vi "Autonomous Independent.vi"() -> ()   [LabVIEW 2017]
doc: "This VI is called when autonomous begins, and will automatically be terminated when autonomous ends. You can carry out timed or sensor driven robot movement independently without needing to return to the caller."
uses:
  <vilib>/Rock Robotics/WPI/RobotDrive/WPI_RobotDriveMecanumDrive_Cartesian.vi
  Robot Global Data.vi
  <vilib>/Rock Robotics/WPI/ThirdParty/Sensors/ADIS16448 IMU/ADIS16448_IMU.lvlib
  <vilib>/Rock Robotics/Network Tables/NT Read String.vi
panel:
  in  "secondTurnAngle":dbl
  in  "distPinceHigh":dbl
  in  "pinceRaiseSpeed":dbl
  in  "pinceLowerSpeed":dbl
  in  "distPinceLow 1":dbl
  in  "angleWall":dbl=-48.0
  in  "angleFloor":dbl=-2.0
  in  "angleRamp":dbl=-7.0
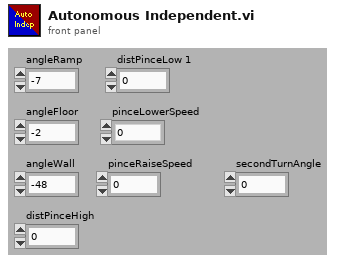
[diagram p1: front panel]
types:
  T1 = typedef "WPI_RobotDriveDevRef.ctl" = cluster{"DevStatus":errorcluster, "Motors[]":T2[], "Square Inputs":bool, "Max Output":dbl}
  T2 = typedef "WPI_MotorControlDeviceRef.ctl" = cluster{"DeviceStatus":errorcluster, "Type":T3, "PWM":cluster{"PWM Channel":T4, "DeadBand":T5}, "CAN":cluster{"Device Number":u8, "SetOutput VI Ref":variant, "GetOutput VI Ref":variant, "Enable VI Ref":variant, "Disable VI Ref":variant, "Data":variant}, "Invert":bool, "DIO PWM":cluster{"PWM \"Enable\" Channel":T4, "DIOChannel":T6, "PWM Rate":dbl}}
  T3 = typedef "WPI_MotorControlType.ctl" = enum16{"PWM", "CAN", "DIO PWM"}
  T4 = typedef "FPGA_DIOPWMChannel.ctl" = enum8{"PWM 0", "PWM 1", "PWM 2", "PWM 3", "PWM 4", "PWM 5", "PWM 6", "PWM 7", "PWM 8", "PWM 9", "PWM MXP 0", "PWM MXP 1", "PWM MXP 2", "PWM MXP 3", "PWM MXP 4", "PWM MXP 5", "PWM MXP 6", "PWM MXP 7", "PWM MXP 8", "PWM MXP 9", "Invalid"}
  T5 = typedef "WPI_PWMDeadband.ctl" = cluster{"Name":string, "maxPositivePwm":i32, "minPositivePwm":i32, "centerPwm":i32, "maxNegativePwm":i32, "minNegativePwm":i32, "angularRange":u16}
  T6 = typedef "FPGA_DIOChannel.ctl" = enum8{"DIO 0", "DIO 1", "DIO 2", "DIO 3", "DIO 4", "DIO 5", "DIO 6", "DIO 7", "DIO 8", "DIO 9", "DIO MXP 0", "DIO MXP 1", "DIO MXP 2", "DIO MXP 3", "DIO MXP 4", "DIO MXP 5", "DIO MXP 6", "DIO MXP 7", "DIO MXP 8", "DIO MXP 9", "DIO MXP 10", "DIO MXP 11", "DIO MXP 12", "DIO MXP 13", "DIO MXP 14", "DIO MXP 15", "SPI Port CS1", "SPI Port CS2", "SPI Port CS3", "SPI Port MISO", "SPI Port MOSI", "Invalid"}
  T7 = typedef "ADIS16448_IMU.lvlib/ADI_IMU_ADIS16448_IMUDevRef.ctl" = cluster{"DevStatus":errorcluster, "Handle":i32, "SPI Bus":T8, "Device Found":bool, "Device Ready":bool, "Yaw Axis":enum16{"X", "Y", "Z"}, "AHRS Algorithm":enum16{"Complementary", "Madgwick"}, "Serial":u16, "Lot ID 2":u16, "Lot ID 1":u16, "Bytes Per Sample":u16, "Calibrate On Open?":bool}
  T8 = typedef "spi_bus.ctl" = enum16{"SPI On-Board, CS0", "SPI On-Board, CS1", "SPI On-Board, CS2", "SPI On-Board, CS3", "SPI MXP", "Invalid"}
  T9 = typedef "WPI_EncoderDevRef.ctl" = cluster{"DevStatus":errorcluster, "EncoderIndex":T10, "CounterIndex":T11, "DistancePerCount":dbl, "Decoding Type":T12}
  T10 = typedef "FPGA_EncoderIdx.ctl" = enum8{"Enc 0", "Enc 1", "Enc 2", "Enc 3", "Enc 4", "Enc 5", "Enc 6", "Enc 7", "Invalid"}
  T11 = typedef "FPGA_CounterCtrSystemIndex.ctl" = enum8{"Ctr 0", "Ctr 1", "Ctr 2", "Ctr 3", "Ctr 4", "Ctr 5", "Ctr 6", "Ctr 7", "Invalid"}
  T12 = typedef "WPI_EncoderType.ctl" = enum16{"1x", "2x", "4x"}
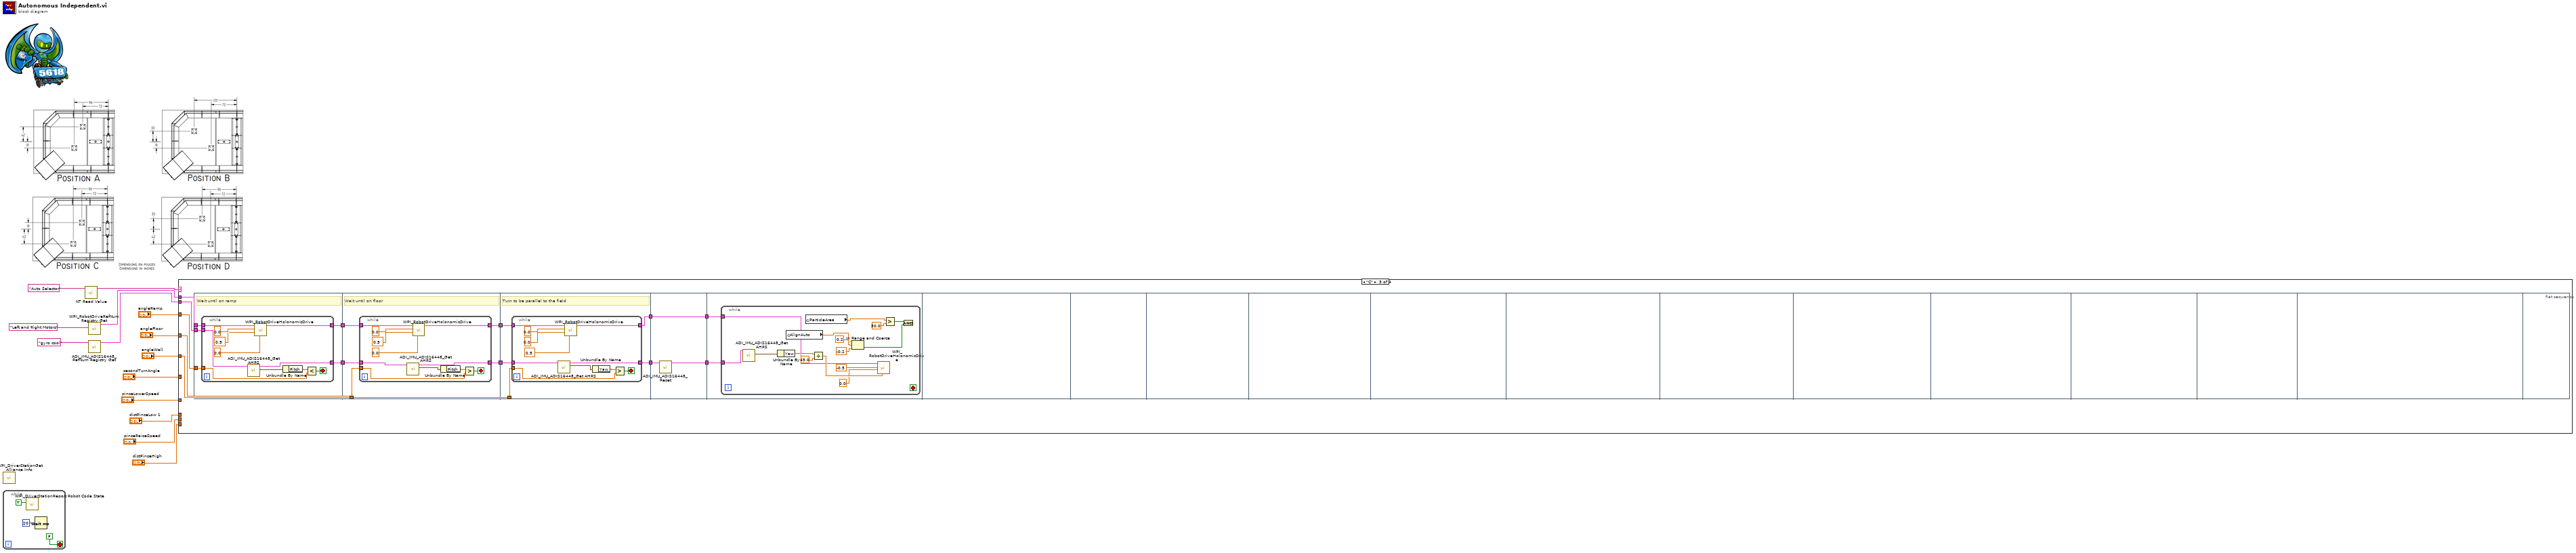
[diagram p0: block diagram]
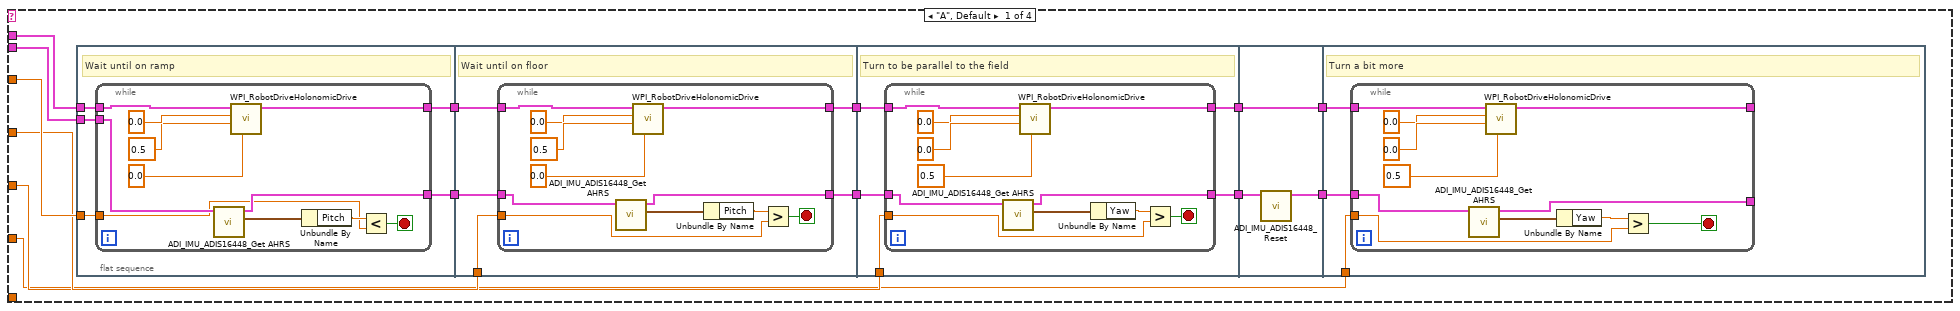
[diagram p2: hidden frame]
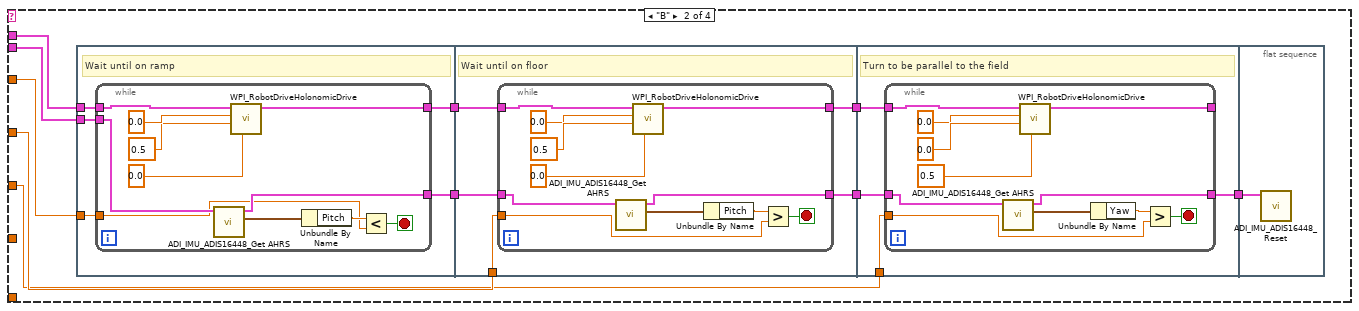
[diagram p3: hidden frame]
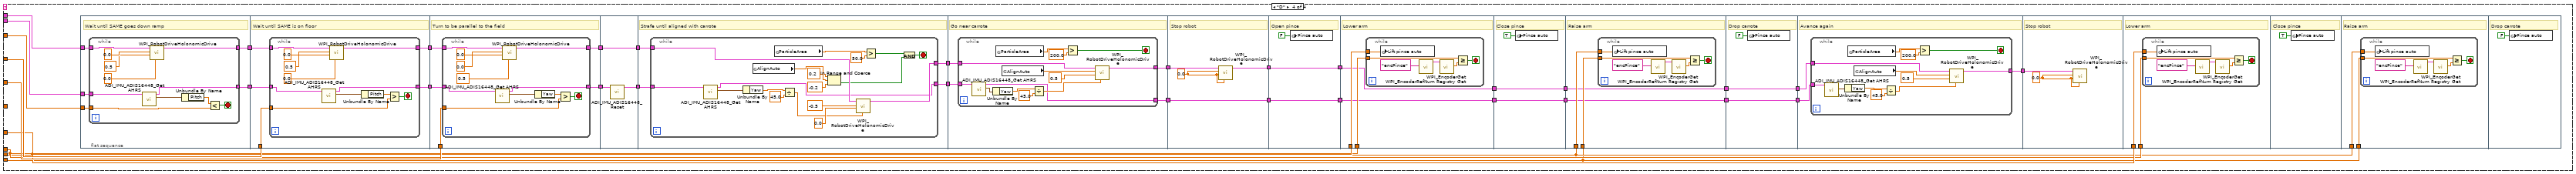
[diagram p4: hidden frame]
diagram:
  n1 = call <vilib>:"WPI_DriverStationGet Alliance Info.vi"() -> ()  [unwired: 12 out]
  n2 = while {
    stop <- FALSE stop-if-true
    n3 = call <vilib>:"WPI_DriverStationReport Robot Code State.vi"("Autonomous"=TRUE) -> ()  [unwired: 10 in, 1 out]
    n4 = Wait (ms)(milliseconds to wait=u32 20) -> ()  [unwired: 1 out]
  }
  n5 = call-poly <vilib>:"NT Read Value.vi"("Name"="Auto Selector") -> ("String"=w13:string)  [unwired: 9 in, 1 out]
  n6 = call <vilib>:"WPI_RobotDriveRefNum Registry Get.vi"("refnum name"="Left and Right Motors") -> ("RobotDriveDevRef"=w11:T1)  [unwired: 9 in, 1 out]
  n7 = call <vilib>:"ADI_IMU_ADIS16448_RefNum Registry Get.vi"("refnum name"="gyro cool") -> ("ADI IMU DevRef"=w9:T7)  [unwired: 9 in, 1 out]
  n8 = case shown="\"C\"" w13 {
    tunnel: w11 -> [w29 w102 w163 w269]
    tunnel: w9 -> [w30 w101 w162 w266]
    tunnel: "angleRamp" -> [w31 w100 w161 w261]
    tunnel: "angleFloor" -> [w28 w99 w160 w260]
    tunnel: "angleWall" -> [w25 w98 w159 w259]
    tunnel: "distPinceLow 1" -> [_ _ _ w243]
    tunnel: "pinceLowerSpeed" -> [_ _ _ w244]
    tunnel: "pinceRaiseSpeed" -> [_ _ _ w242]
    tunnel: "distPinceHigh" -> [_ _ _ w241]
    tunnel: "secondTurnAngle" -> [w18 _ _ _]
    frame "A", Default {
      n9 = flat-sequence {
        tunnel: w31 -> [w36]
        tunnel: w30 -> [w35]
        tunnel: w29 -> [w34]
        tunnel: [w33] -> w27
        tunnel: [w32] -> w26
        tunnel: w28 -> [w52]
        tunnel: w27 -> [w51]
        tunnel: w26 -> [w50]
        tunnel: [w49] -> w24
        tunnel: [w48] -> w23
        tunnel: w25 -> [w68]
        tunnel: w24 -> [w67]
        tunnel: w23 -> [w66]
        tunnel: [w65] -> w22
        tunnel: [w64] -> w19
        tunnel: w22 -> [w82]
        tunnel: [w81] -> w21
        tunnel: [w80] -> w20
        tunnel: w19 -> [w80]
        tunnel: w21 -> [w85]
        tunnel: w20 -> [w84]
        tunnel: w18 -> [w83]
        frame #0 {
          # "Wait until on ramp"
          n10 = while {
            tunnel: w34 -> [w47]
            tunnel: [w43] -> w33
            tunnel: w35 -> [w41]
            tunnel: [w38] -> w32
            tunnel: w36 -> [w37]
            stop <- w39 stop-if-true
            n11 = call <vilib>:"ADI_IMU_ADIS16448_Get AHRS.vi"("ADI IMU DevRef"=w41) -> ("IMU AHRS Out"=w42:cluster{"Pitch":dbl, "Roll":dbl, "Yaw":dbl}, "ADI IMU DevRef Out"=w38:T7)  [unwired: 7 in, 2 out]
            n12 = call-poly <vilib>:"WPI_RobotDriveHolonomicDrive.vi"("Rotation"=0.0, "Y"=0.5, "X"=0.0, "RobotDriveDevRef"=w47) -> ("RobotDriveDevRef"=w43:T1)  [unwired: 5 in, 2 out]
            n13 = Unbundle By Name(w42) -> ("Pitch"=w40:dbl)
            n14 = Less?(x=w40, y=w37) -> (x < y?=w39:bool)
          }
        }
        frame #1 {
          # "Wait until on floor"
          n15 = while {
            tunnel: w51 -> [w60]
            tunnel: [w59] -> w48
            tunnel: w50 -> [w56]
            tunnel: [w54] -> w49
            tunnel: w52 -> [w53]
            stop <- w55 stop-if-true
            n16 = call <vilib>:"ADI_IMU_ADIS16448_Get AHRS.vi"("ADI IMU DevRef"=w56) -> ("IMU AHRS Out"=w58:cluster{"Pitch":dbl, "Roll":dbl, "Yaw":dbl}, "ADI IMU DevRef Out"=w54:T7)  [unwired: 7 in, 2 out]
            n17 = call-poly <vilib>:"WPI_RobotDriveHolonomicDrive.vi"("Rotation"=0.0, "Y"=0.5, "X"=0.0, "RobotDriveDevRef"=w60) -> ("RobotDriveDevRef"=w59:T1)  [unwired: 5 in, 2 out]
            n18 = Unbundle By Name(w58) -> ("Pitch"=w57:dbl)
            n19 = Greater?(x=w57, y=w53) -> (0:w55:bool)
          }
        }
        frame #2 {
          # "Turn to be parallel to the field"
          n20 = while {
            tunnel: w66 -> [w78]
            tunnel: [w77] -> w64
            tunnel: w67 -> [w74]
            tunnel: [w70] -> w65
            tunnel: w68 -> [w69]
            stop <- w73 stop-if-true
            n21 = call <vilib>:"ADI_IMU_ADIS16448_Get AHRS.vi"("ADI IMU DevRef"=w74) -> ("IMU AHRS Out"=w76:cluster{"Pitch":dbl, "Roll":dbl, "Yaw":dbl}, "ADI IMU DevRef Out"=w70:T7)  [unwired: 7 in, 2 out]
            n22 = call-poly <vilib>:"WPI_RobotDriveHolonomicDrive.vi"("Rotation"=0.5, "Y"=0.0, "X"=0.0, "RobotDriveDevRef"=w78) -> ("RobotDriveDevRef"=w77:T1)  [unwired: 5 in, 2 out]
            n23 = Unbundle By Name(w76) -> ("Yaw"=w75:dbl)
            n24 = Greater?(x=w75, y=w69) -> (0:w73:bool)
          }
        }
        frame #3 {
          n25 = call <vilib>:"ADI_IMU_ADIS16448_Reset.vi"("ADI IMU DevRef"=w82) -> ("ADI IMU DevRef Out"=w81:T7)  [unwired: 9 in, 1 out]
        }
        frame #4 {
          # "Turn a bit more"
          n26 = while {
            tunnel: w84 -> [w95]
            tunnel: [w94] -> _
            tunnel: w85 -> [w91]
            tunnel: [w87] -> _
            tunnel: w83 -> [w86]
            stop <- w90 stop-if-true
            n27 = call <vilib>:"ADI_IMU_ADIS16448_Get AHRS.vi"("ADI IMU DevRef"=w91) -> ("IMU AHRS Out"=w93:cluster{"Pitch":dbl, "Roll":dbl, "Yaw":dbl}, "ADI IMU DevRef Out"=w87:T7)  [unwired: 7 in, 2 out]
            n28 = call-poly <vilib>:"WPI_RobotDriveHolonomicDrive.vi"("Rotation"=0.5, "Y"=0.0, "X"=0.0, "RobotDriveDevRef"=w95) -> ("RobotDriveDevRef"=w94:T1)  [unwired: 5 in, 2 out]
            n29 = Unbundle By Name(w93) -> ("Yaw"=w92:dbl)
            n30 = Greater?(x=w92, y=w86) -> (0:w90:bool)
          }
        }
      }
    }
    frame "B" {
      n31 = flat-sequence {
        tunnel: w100 -> [w111]
        tunnel: w101 -> [w110]
        tunnel: w102 -> [w109]
        tunnel: [w108] -> w106
        tunnel: [w107] -> w105
        tunnel: w99 -> [w127]
        tunnel: w106 -> [w126]
        tunnel: w105 -> [w125]
        tunnel: [w124] -> w104
        tunnel: [w123] -> w103
        tunnel: w98 -> [w142]
        tunnel: w104 -> [w141]
        tunnel: w103 -> [w140]
        tunnel: [w139] -> w97
        tunnel: w97 -> [w154]
        frame #0 {
          # "Wait until on ramp"
          n32 = while {
            tunnel: w109 -> [w122]
            tunnel: [w118] -> w108
            tunnel: w110 -> [w116]
            tunnel: [w113] -> w107
            tunnel: w111 -> [w112]
            stop <- w114 stop-if-true
            n33 = call <vilib>:"ADI_IMU_ADIS16448_Get AHRS.vi"("ADI IMU DevRef"=w116) -> ("IMU AHRS Out"=w117:cluster{"Pitch":dbl, "Roll":dbl, "Yaw":dbl}, "ADI IMU DevRef Out"=w113:T7)  [unwired: 7 in, 2 out]
            n34 = call-poly <vilib>:"WPI_RobotDriveHolonomicDrive.vi"("Rotation"=0.0, "Y"=0.5, "X"=0.0, "RobotDriveDevRef"=w122) -> ("RobotDriveDevRef"=w118:T1)  [unwired: 5 in, 2 out]
            n35 = Unbundle By Name(w117) -> ("Pitch"=w115:dbl)
            n36 = Less?(x=w115, y=w112) -> (x < y?=w114:bool)
          }
        }
        frame #1 {
          # "Wait until on floor"
          n37 = while {
            tunnel: w126 -> [w135]
            tunnel: [w134] -> w123
            tunnel: w125 -> [w131]
            tunnel: [w129] -> w124
            tunnel: w127 -> [w128]
            stop <- w130 stop-if-true
            n38 = call <vilib>:"ADI_IMU_ADIS16448_Get AHRS.vi"("ADI IMU DevRef"=w131) -> ("IMU AHRS Out"=w133:cluster{"Pitch":dbl, "Roll":dbl, "Yaw":dbl}, "ADI IMU DevRef Out"=w129:T7)  [unwired: 7 in, 2 out]
            n39 = call-poly <vilib>:"WPI_RobotDriveHolonomicDrive.vi"("Rotation"=0.0, "Y"=0.5, "X"=0.0, "RobotDriveDevRef"=w135) -> ("RobotDriveDevRef"=w134:T1)  [unwired: 5 in, 2 out]
            n40 = Unbundle By Name(w133) -> ("Pitch"=w132:dbl)
            n41 = Greater?(x=w132, y=w128) -> (0:w130:bool)
          }
        }
        frame #2 {
          # "Turn to be parallel to the field"
          n42 = while {
            tunnel: w140 -> [w152]
            tunnel: [w151] -> _
            tunnel: w141 -> [w148]
            tunnel: [w144] -> w139
            tunnel: w142 -> [w143]
            stop <- w147 stop-if-true
            n43 = call <vilib>:"ADI_IMU_ADIS16448_Get AHRS.vi"("ADI IMU DevRef"=w148) -> ("IMU AHRS Out"=w150:cluster{"Pitch":dbl, "Roll":dbl, "Yaw":dbl}, "ADI IMU DevRef Out"=w144:T7)  [unwired: 7 in, 2 out]
            n44 = call-poly <vilib>:"WPI_RobotDriveHolonomicDrive.vi"("Rotation"=0.5, "Y"=0.0, "X"=0.0, "RobotDriveDevRef"=w152) -> ("RobotDriveDevRef"=w151:T1)  [unwired: 5 in, 2 out]
            n45 = Unbundle By Name(w150) -> ("Yaw"=w149:dbl)
            n46 = Greater?(x=w149, y=w143) -> (0:w147:bool)
          }
        }
        frame #3 {
          n47 = call <vilib>:"ADI_IMU_ADIS16448_Reset.vi"("ADI IMU DevRef"=w154) -> ()  [unwired: 9 in, 2 out]
        }
      }
    }
    frame "C" {
      n48 = flat-sequence {
        tunnel: w161 -> [w172]
        tunnel: w162 -> [w171]
        tunnel: w163 -> [w170]
        tunnel: [w169] -> w167
        tunnel: [w168] -> w166
        tunnel: w160 -> [w188]
        tunnel: w167 -> [w187]
        tunnel: w166 -> [w186]
        tunnel: [w185] -> w165
        tunnel: [w184] -> w164
        tunnel: w159 -> [w204]
        tunnel: w165 -> [w203]
        tunnel: w164 -> [w202]
        tunnel: [w201] -> w158
        tunnel: [w200] -> w155
        tunnel: w158 -> [w218]
        tunnel: [w217] -> w157
        tunnel: [w216] -> w156
        tunnel: w155 -> [w216]
        tunnel: w157 -> [w220]
        tunnel: w156 -> [w219]
        frame #0 {
          # "Wait until on ramp"
          n49 = while {
            tunnel: w170 -> [w183]
            tunnel: [w179] -> w169
            tunnel: w171 -> [w177]
            tunnel: [w174] -> w168
            tunnel: w172 -> [w173]
            stop <- w175 stop-if-true
            n50 = call <vilib>:"ADI_IMU_ADIS16448_Get AHRS.vi"("ADI IMU DevRef"=w177) -> ("IMU AHRS Out"=w178:cluster{"Pitch":dbl, "Roll":dbl, "Yaw":dbl}, "ADI IMU DevRef Out"=w174:T7)  [unwired: 7 in, 2 out]
            n51 = call-poly <vilib>:"WPI_RobotDriveHolonomicDrive.vi"("Rotation"=0.0, "Y"=0.5, "X"=0.0, "RobotDriveDevRef"=w183) -> ("RobotDriveDevRef"=w179:T1)  [unwired: 5 in, 2 out]
            n52 = Unbundle By Name(w178) -> ("Pitch"=w176:dbl)
            n53 = Less?(x=w176, y=w173) -> (x < y?=w175:bool)
          }
        }
        frame #1 {
          # "Wait until on floor"
          n54 = while {
            tunnel: w187 -> [w196]
            tunnel: [w195] -> w184
            tunnel: w186 -> [w192]
            tunnel: [w190] -> w185
            tunnel: w188 -> [w189]
            stop <- w191 stop-if-true
            n55 = call <vilib>:"ADI_IMU_ADIS16448_Get AHRS.vi"("ADI IMU DevRef"=w192) -> ("IMU AHRS Out"=w194:cluster{"Pitch":dbl, "Roll":dbl, "Yaw":dbl}, "ADI IMU DevRef Out"=w190:T7)  [unwired: 7 in, 2 out]
            n56 = call-poly <vilib>:"WPI_RobotDriveHolonomicDrive.vi"("Rotation"=0.0, "Y"=0.5, "X"=0.0, "RobotDriveDevRef"=w196) -> ("RobotDriveDevRef"=w195:T1)  [unwired: 5 in, 2 out]
            n57 = Unbundle By Name(w194) -> ("Pitch"=w193:dbl)
            n58 = Greater?(x=w193, y=w189) -> (0:w191:bool)
          }
        }
        frame #2 {
          # "Turn to be parallel to the field"
          n59 = while {
            tunnel: w202 -> [w214]
            tunnel: [w213] -> w200
            tunnel: w203 -> [w210]
            tunnel: [w206] -> w201
            tunnel: w204 -> [w205]
            stop <- w209 stop-if-true
            n60 = call <vilib>:"ADI_IMU_ADIS16448_Get AHRS.vi"("ADI IMU DevRef"=w210) -> ("IMU AHRS Out"=w212:cluster{"Pitch":dbl, "Roll":dbl, "Yaw":dbl}, "ADI IMU DevRef Out"=w206:T7)  [unwired: 7 in, 2 out]
            n61 = call-poly <vilib>:"WPI_RobotDriveHolonomicDrive.vi"("Rotation"=0.5, "Y"=0.0, "X"=0.0, "RobotDriveDevRef"=w214) -> ("RobotDriveDevRef"=w213:T1)  [unwired: 5 in, 2 out]
            n62 = Unbundle By Name(w212) -> ("Yaw"=w211:dbl)
            n63 = Greater?(x=w211, y=w205) -> (0:w209:bool)
          }
        }
        frame #3 {
          n64 = call <vilib>:"ADI_IMU_ADIS16448_Reset.vi"("ADI IMU DevRef"=w218) -> ("ADI IMU DevRef Out"=w217:T7)  [unwired: 9 in, 1 out]
        }
        frame #4 {
          n65 = while {
            tunnel: w220 -> [w222]
            tunnel: w219 -> [w221]
            stop <- _ stop-if-true
            n66 = call <vilib>:"ADI_IMU_ADIS16448_Get AHRS.vi"("ADI IMU DevRef"=w222) -> ("IMU AHRS Out"=w233:cluster{"Pitch":dbl, "Roll":dbl, "Yaw":dbl})  [unwired: 7 in, 3 out]
            n67 = Unbundle By Name(w233) -> ("Yaw"=w235:dbl)
            n68 = global read "Robot Global Data.vi" "AlignAuto"() -> (w232:dbl)
            n69 = global read "Robot Global Data.vi" "ParticleArea"() -> (w229:dbl)
            n70 = Divide(x=w235, y=45.0) -> (x/y=w234:dbl)
            n71 = In Range and Coerce(upper limit=0.2, x=w232, lower limit=-0.2) -> (In Range?=w231:bool)  [unwired: 1 out]
            n72 = call-poly <vilib>:"WPI_RobotDriveHolonomicDrive.vi"("Rotation"=w234, "Y"=0.0, "X"=-0.5, "RobotDriveDevRef"=w221) -> ()  [unwired: 5 in, 3 out]
            n73 = Greater?(x=w229, y=50.0) -> (0:w230:bool)
            n74 = And(x=w230, y=w231) -> ()  [unwired: 1 out]
          }
        }
        frame #5 {
        }
        frame #6 {
        }
        frame #7 {
        }
        frame #8 {
        }
        frame #9 {
        }
        frame #10 {
        }
        frame #11 {
        }
        frame #12 {
        }
        frame #13 {
        }
        frame #14 {
        }
        frame #15 {
        }
        frame #16 {
        }
        frame #17 {
        }
      }
    }
    frame "D" {
      n75 = flat-sequence {
        tunnel: w269 -> [w274]
        tunnel: [w273] -> w268
        tunnel: w266 -> [w272]
        tunnel: [w271] -> w265
        tunnel: w261 -> [w270]
        tunnel: w268 -> [w290]
        tunnel: [w289] -> w267
        tunnel: w265 -> [w288]
        tunnel: [w287] -> w264
        tunnel: w260 -> [w286]
        tunnel: w267 -> [w306]
        tunnel: [w305] -> w258
        tunnel: w264 -> [w304]
        tunnel: [w303] -> w256
        tunnel: w259 -> [w302]
        tunnel: w258 -> [w320]
        tunnel: [w320] -> w257
        tunnel: w256 -> [w319]
        tunnel: [w318] -> w255
        tunnel: w257 -> [w324]
        tunnel: [w322] -> w263
        tunnel: w255 -> [w323]
        tunnel: [w321] -> w262
        tunnel: w263 -> [w346]
        tunnel: w262 -> [w345]
        tunnel: [w344] -> w240
        tunnel: [w343] -> w238
        tunnel: w240 -> [w362]
        tunnel: [w361] -> w239
        tunnel: w238 -> [w363]
        tunnel: [w363] -> w237
        tunnel: [w366] -> w252
        tunnel: w239 -> [w366]
        tunnel: [w365] -> w249
        tunnel: w237 -> [w365]
        tunnel: w243 -> [w370]
        tunnel: w244 -> [w369]
        tunnel: [w368] -> w253
        tunnel: w252 -> [w368]
        tunnel: [w367] -> w250
        tunnel: w249 -> [w367]
        tunnel: [w378] -> w254
        tunnel: w253 -> [w378]
        tunnel: [w377] -> w251
        tunnel: w250 -> [w377]
        tunnel: w242 -> [w383]
        tunnel: w241 -> [w382]
        tunnel: [w381] -> w248
        tunnel: w254 -> [w381]
        tunnel: [w380] -> w246
        tunnel: w251 -> [w380]
        tunnel: w248 -> [w392]
        tunnel: [w392] -> w247
        tunnel: w246 -> [w391]
        tunnel: [w391] -> w245
        tunnel: w247 -> [w395]
        tunnel: w245 -> [w394]
        tunnel: [w393] -> w236
        tunnel: w236 -> [w408]
        tunnel: w244 -> [w411]
        tunnel: w243 -> [w410]
        tunnel: w242 -> [w420]
        tunnel: w241 -> [w419]
        frame #0 {
          # "Wait until SAME goes down ramp"
          n76 = while {
            tunnel: w274 -> [w285]
            tunnel: [w281] -> w273
            tunnel: w272 -> [w279]
            tunnel: [w276] -> w271
            tunnel: w270 -> [w275]
            stop <- w277 stop-if-true
            n77 = call <vilib>:"ADI_IMU_ADIS16448_Get AHRS.vi"("ADI IMU DevRef"=w279) -> ("IMU AHRS Out"=w280:cluster{"Pitch":dbl, "Roll":dbl, "Yaw":dbl}, "ADI IMU DevRef Out"=w276:T7)  [unwired: 7 in, 2 out]
            n78 = call-poly <vilib>:"WPI_RobotDriveHolonomicDrive.vi"("Rotation"=0.0, "Y"=0.5, "X"=0.0, "RobotDriveDevRef"=w285) -> ("RobotDriveDevRef"=w281:T1)  [unwired: 5 in, 2 out]
            n79 = Unbundle By Name(w280) -> ("Pitch"=w278:dbl)
            n80 = Less?(x=w278, y=w275) -> (x < y?=w277:bool)
          }
        }
        frame #1 {
          # "Wait until SAME is on floor"
          n81 = while {
            tunnel: w290 -> [w298]
            tunnel: [w297] -> w289
            tunnel: w288 -> [w294]
            tunnel: [w292] -> w287
            tunnel: w286 -> [w291]
            stop <- w293 stop-if-true
            n82 = call <vilib>:"ADI_IMU_ADIS16448_Get AHRS.vi"("ADI IMU DevRef"=w294) -> ("IMU AHRS Out"=w296:cluster{"Pitch":dbl, "Roll":dbl, "Yaw":dbl}, "ADI IMU DevRef Out"=w292:T7)  [unwired: 7 in, 2 out]
            n83 = call-poly <vilib>:"WPI_RobotDriveHolonomicDrive.vi"("Rotation"=0.0, "Y"=0.5, "X"=0.0, "RobotDriveDevRef"=w298) -> ("RobotDriveDevRef"=w297:T1)  [unwired: 5 in, 2 out]
            n84 = Unbundle By Name(w296) -> ("Pitch"=w295:dbl)
            n85 = Greater?(x=w295, y=w291) -> (0:w293:bool)
          }
        }
        frame #2 {
          # "Turn to be parallel to the field"
          n86 = while {
            tunnel: w306 -> [w316]
            tunnel: [w315] -> w305
            tunnel: w304 -> [w312]
            tunnel: [w308] -> w303
            tunnel: w302 -> [w307]
            stop <- w311 stop-if-true
            n87 = call <vilib>:"ADI_IMU_ADIS16448_Get AHRS.vi"("ADI IMU DevRef"=w312) -> ("IMU AHRS Out"=w314:cluster{"Pitch":dbl, "Roll":dbl, "Yaw":dbl}, "ADI IMU DevRef Out"=w308:T7)  [unwired: 7 in, 2 out]
            n88 = call-poly <vilib>:"WPI_RobotDriveHolonomicDrive.vi"("Rotation"=0.5, "Y"=0.0, "X"=0.0, "RobotDriveDevRef"=w316) -> ("RobotDriveDevRef"=w315:T1)  [unwired: 5 in, 2 out]
            n89 = Unbundle By Name(w314) -> ("Yaw"=w313:dbl)
            n90 = Greater?(x=w313, y=w307) -> (0:w311:bool)
          }
        }
        frame #3 {
          n91 = call <vilib>:"ADI_IMU_ADIS16448_Reset.vi"("ADI IMU DevRef"=w319) -> ("ADI IMU DevRef Out"=w318:T7)  [unwired: 9 in, 1 out]
        }
        frame #4 {
          # "Strafe until aligned with carrote"
          n92 = while {
            tunnel: w324 -> [w340]
            tunnel: w323 -> [w331]
            tunnel: [w328] -> w322
            tunnel: [w327] -> w321
            stop <- w336 stop-if-true
            n93 = call <vilib>:"ADI_IMU_ADIS16448_Get AHRS.vi"("ADI IMU DevRef"=w331) -> ("IMU AHRS Out"=w330:cluster{"Pitch":dbl, "Roll":dbl, "Yaw":dbl}, "ADI IMU DevRef Out"=w327:T7)  [unwired: 7 in, 2 out]
            n94 = Unbundle By Name(w330) -> ("Yaw"=w326:dbl)
            n95 = global read "Robot Global Data.vi" "AlignAuto"() -> (w334:dbl)
            n96 = global read "Robot Global Data.vi" "ParticleArea"() -> (w339:dbl)
            n97 = Divide(x=w326, y=45.0) -> (x/y=w329:dbl)
            n98 = In Range and Coerce(upper limit=0.2, x=w334, lower limit=-0.2) -> (In Range?=w335:bool)  [unwired: 1 out]
            n99 = call-poly <vilib>:"WPI_RobotDriveHolonomicDrive.vi"("Rotation"=w329, "Y"=0.0, "X"=-0.5, "RobotDriveDevRef"=w340) -> ("RobotDriveDevRef"=w328:T1)  [unwired: 5 in, 2 out]
            n100 = Greater?(x=w339, y=50.0) -> (0:w337:bool)
            n101 = And(x=w337, y=w335) -> (x .and. y?=w336:bool)
          }
        }
        frame #5 {
          # "Go near carrote"
          n102 = while {
            tunnel: w346 -> [w358]
            tunnel: w345 -> [w355]
            tunnel: [w348] -> w344
            tunnel: [w347] -> w343
            stop <- w350 stop-if-true
            n103 = call <vilib>:"ADI_IMU_ADIS16448_Get AHRS.vi"("ADI IMU DevRef"=w355) -> ("IMU AHRS Out"=w354:cluster{"Pitch":dbl, "Roll":dbl, "Yaw":dbl}, "ADI IMU DevRef Out"=w347:T7)  [unwired: 7 in, 2 out]
            n104 = Unbundle By Name(w354) -> ("Yaw"=w352:dbl)
            n105 = global read "Robot Global Data.vi" "ParticleArea"() -> (w357:dbl)
            n106 = global read "Robot Global Data.vi" "AlignAuto"() -> (w349:dbl)
            n107 = Divide(x=w352, y=45.0) -> (x/y=w353:dbl)
            n108 = Greater?(x=w357, y=200.0) -> (0:w350:bool)
            n109 = call-poly <vilib>:"WPI_RobotDriveHolonomicDrive.vi"("Rotation"=w353, "Y"=0.5, "X"=w349, "RobotDriveDevRef"=w358) -> ("RobotDriveDevRef"=w348:T1)  [unwired: 5 in, 2 out]
          }
        }
        frame #6 {
          w360 = 0.0 ("X")
          # "Stop robot"
          n110 = call-poly <vilib>:"WPI_RobotDriveHolonomicDrive.vi"("Rotation"=w360, "Y"=w360, "X"=w360, "RobotDriveDevRef"=w362) -> ("RobotDriveDevRef"=w361:T1)  [unwired: 5 in, 2 out]
        }
        frame #7 {
          # "Open pince"
          n111 = global write "Robot Global Data.vi" "Pince auto"(FALSE ("Pince auto")) -> ()
        }
        frame #8 {
          # "Lower arm"
          n112 = while {
            tunnel: w370 -> [w372]
            tunnel: w369 -> [w371]
            stop <- w373 stop-if-true
            n113 = global write "Robot Global Data.vi" "Lift pince auto"(w371) -> ()
            n114 = call <vilib>:"WPI_EncoderRefNum Registry Get.vi"("refnum name"="encPince") -> ("EncoderDevRef"=w376:T9)  [unwired: 9 in, 1 out]
            n115 = call <vilib>:"WPI_EncoderGet.vi"("EncoderDevRef"=w376) -> ("Distance"=w374:dbl)  [unwired: 5 in, 5 out]
            n116 = Greater Or Equal?(x=w372, y=w374) -> (x >= y?=w373:bool)
          }
        }
        frame #9 {
          # "Close pince"
          n117 = global write "Robot Global Data.vi" "Pince auto"(TRUE ("Pince auto")) -> ()
        }
        frame #10 {
          # "Raise arm"
          n118 = while {
            tunnel: w383 -> [w385]
            tunnel: w382 -> [w384]
            stop <- w386 stop-if-true
            n119 = global write "Robot Global Data.vi" "Lift pince auto"(w385) -> ()
            n120 = call <vilib>:"WPI_EncoderRefNum Registry Get.vi"("refnum name"="encPince") -> ("EncoderDevRef"=w389:T9)  [unwired: 9 in, 1 out]
            n121 = call <vilib>:"WPI_EncoderGet.vi"("EncoderDevRef"=w389) -> ("Distance"=w387:dbl)  [unwired: 5 in, 5 out]
            n122 = Greater Or Equal?(x=w384, y=w387) -> (x >= y?=w386:bool)
          }
        }
        frame #11 {
          # "Drop carrote"
          n123 = global write "Robot Global Data.vi" "Pince auto"(FALSE ("Pince auto")) -> ()
        }
        frame #12 {
          # "Avance again"
          n124 = while {
            tunnel: w395 -> [w406]
            tunnel: w394 -> [w403]
            tunnel: [w396] -> w393
            stop <- w398 stop-if-true
            n125 = call <vilib>:"ADI_IMU_ADIS16448_Get AHRS.vi"("ADI IMU DevRef"=w403) -> ("IMU AHRS Out"=w402:cluster{"Pitch":dbl, "Roll":dbl, "Yaw":dbl})  [unwired: 7 in, 3 out]
            n126 = Unbundle By Name(w402) -> ("Yaw"=w400:dbl)
            n127 = global read "Robot Global Data.vi" "ParticleArea"() -> (w405:dbl)
            n128 = global read "Robot Global Data.vi" "AlignAuto"() -> (w397:dbl)
            n129 = Divide(x=w400, y=45.0) -> (x/y=w401:dbl)
            n130 = Greater?(x=w405, y=200.0) -> (0:w398:bool)
            n131 = call-poly <vilib>:"WPI_RobotDriveHolonomicDrive.vi"("Rotation"=w401, "Y"=0.5, "X"=w397, "RobotDriveDevRef"=w406) -> ("RobotDriveDevRef"=w396:T1)  [unwired: 5 in, 2 out]
          }
        }
        frame #13 {
          w409 = 0.0 ("X")
          # "Stop robot"
          n132 = call-poly <vilib>:"WPI_RobotDriveHolonomicDrive.vi"("Rotation"=w409, "Y"=w409, "X"=w409, "RobotDriveDevRef"=w408) -> ()  [unwired: 5 in, 3 out]
        }
        frame #14 {
          # "Lower arm"
          n133 = while {
            tunnel: w410 -> [w413]
            tunnel: w411 -> [w412]
            stop <- w414 stop-if-true
            n134 = global write "Robot Global Data.vi" "Lift pince auto"(w412) -> ()
            n135 = call <vilib>:"WPI_EncoderRefNum Registry Get.vi"("refnum name"="encPince") -> ("EncoderDevRef"=w417:T9)  [unwired: 9 in, 1 out]
            n136 = call <vilib>:"WPI_EncoderGet.vi"("EncoderDevRef"=w417) -> ("Distance"=w415:dbl)  [unwired: 5 in, 5 out]
            n137 = Greater Or Equal?(x=w413, y=w415) -> (x >= y?=w414:bool)
          }
        }
        frame #15 {
          # "Close pince"
          n138 = global write "Robot Global Data.vi" "Pince auto"(TRUE ("Pince auto")) -> ()
        }
        frame #16 {
          # "Raise arm"
          n139 = while {
            tunnel: w420 -> [w422]
            tunnel: w419 -> [w421]
            stop <- w423 stop-if-true
            n140 = global write "Robot Global Data.vi" "Lift pince auto"(w422) -> ()
            n141 = call <vilib>:"WPI_EncoderRefNum Registry Get.vi"("refnum name"="encPince") -> ("EncoderDevRef"=w426:T9)  [unwired: 9 in, 1 out]
            n142 = call <vilib>:"WPI_EncoderGet.vi"("EncoderDevRef"=w426) -> ("Distance"=w424:dbl)  [unwired: 5 in, 5 out]
            n143 = Greater Or Equal?(x=w421, y=w424) -> (x >= y?=w423:bool)
          }
        }
        frame #17 {
          # "Drop carrote"
          n144 = global write "Robot Global Data.vi" "Pince auto"(FALSE ("Pince auto")) -> ()
        }
      }
    }
  }
